vi "Template Write Parameter File.vi"(6 "Export?":bool, 8 "error in (no error)":errorcluster, 9 "Export Path (\"\")":path, 10 "Parameters (empty)":T3, 11 "Template Record":T1) -> (0 "error out":errorcluster, 2 "Template Record 2":T1, 3 "Files":T2)   [LabVIEW 2011]
uses:
  Addons/internet/utils/keyedarr.llb/Keyed Array.ctl
  Template Record.ctl
  <vilib>/Utility/config.llb/Write Key (String).vi
  <vilib>/Utility/config.llb/NI_LVConfig.lvlib
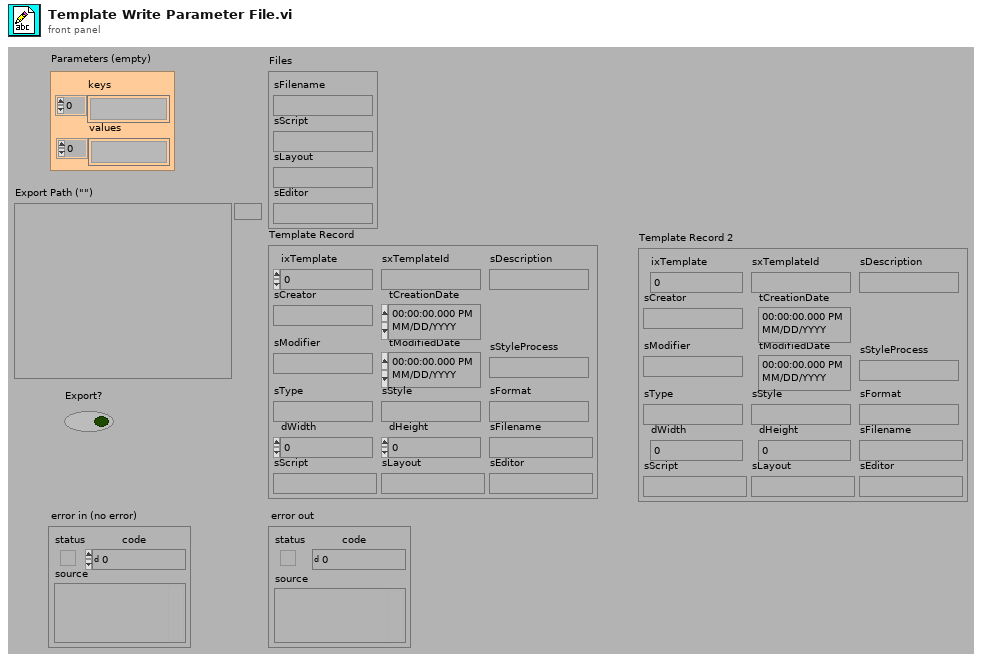
[diagram p1: front panel]
types:
  T1 = typedef "Template Record.ctl" = cluster{"ixTemplate":i32, "sxTemplateId":string, "sDescription":string, "sCreator":string, "tCreationDate":timestamp, "sModifier":string, "tModifiedDate":timestamp, "sType":string, "sStyle":string, "sFormat":string, "dWidth":dbl, "dHeight":dbl, "sFilename":string, "sScript":string, "sLayout":string, "sEditor":string, "sStyleProcess":string}
  T2 = cluster{"sFilename":string, "sScript":string, "sLayout":string, "sEditor":string}
  T3 = typedef "Keyed Array.ctl" = cluster{"keys":string[], "values":string[]}
  T4 = typedef "NI_LVConfig.lvlib/Config Data RefNum.ctl" = refnum<k1>
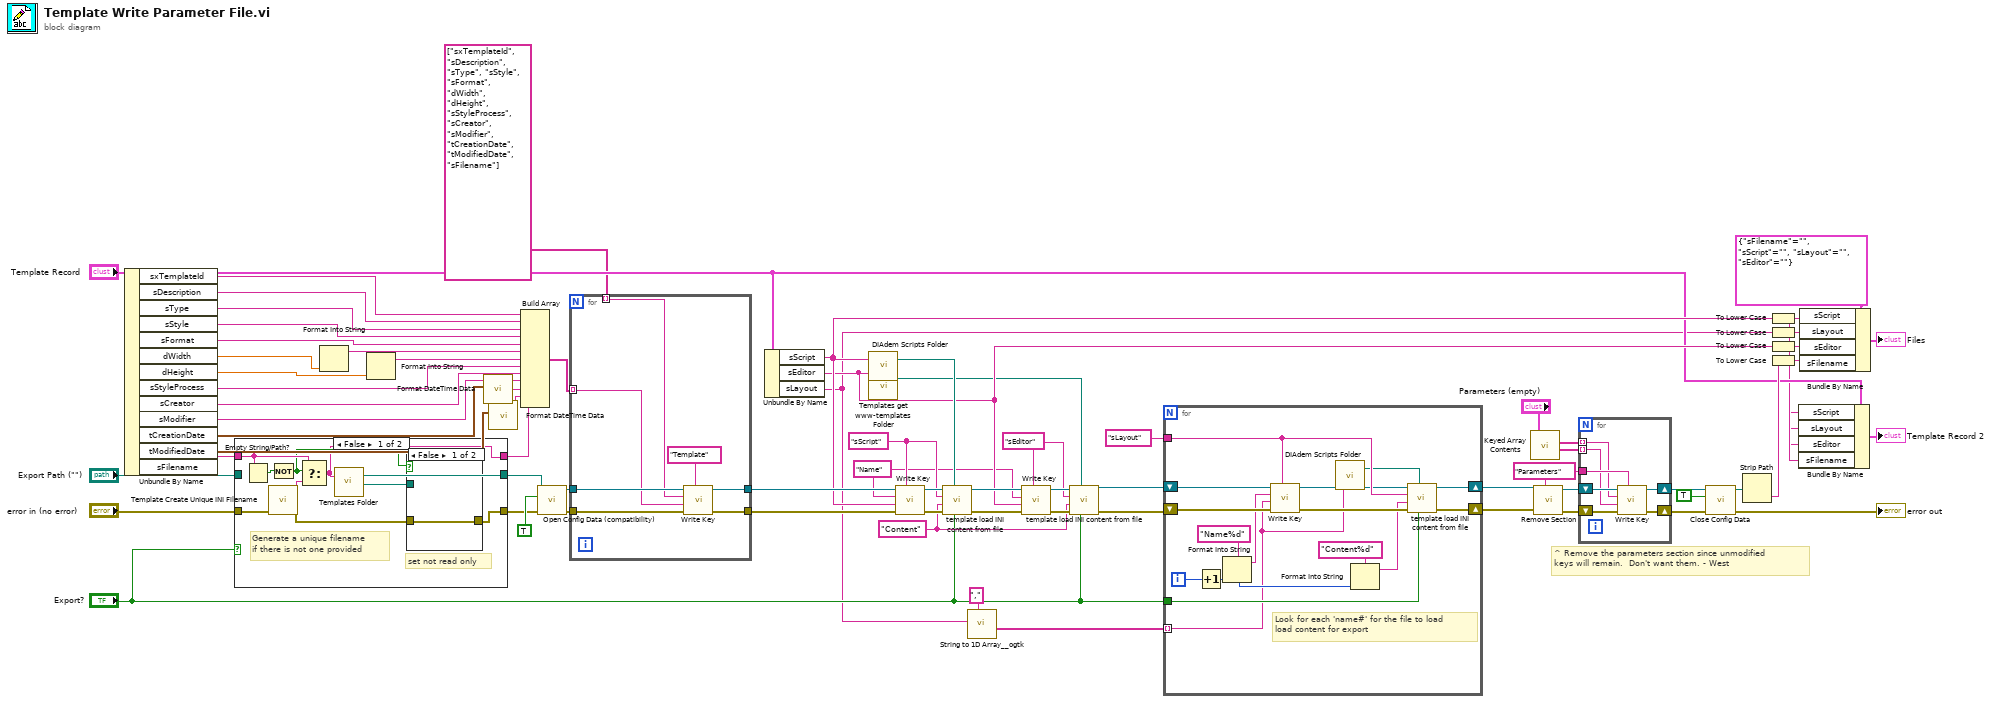
[diagram p0: block diagram]
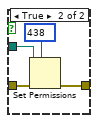
[diagram p2: hidden frame]
diagram:
  w29 = "Content" ("section")
  w40 = "Parameters" ("section")
  w32 = "sEditor" ("section")
  w28 = "Name" ("section")
  w37 = "sScript" ("section")
  # "^ Remove the parameters section since unmodified\nkeys will remain.  Don't want them. - West"
  n1 = Unbundle By Name("Template Record") -> ("sxTemplateId"=w67:string, "sDescription"=w65:string, "sType"=w64:string, "sStyle"=w63:string, "sFormat"=w41:string, "dWidth"=w47:dbl, "dHeight"=w45:dbl, "sStyleProcess"=w12:string, "sCreator"=w10:string, "sModifier"=w9:string, "tCreationDate"=w8:timestamp, "tModifiedDate"=w5:timestamp, "sFilename"=w62:string)
  n2 = case shown="False" "Export?" {
    tunnel: [w74 w89] -> w20
    tunnel: w62 -> [w80 w87]
    tunnel: "error in (no error)" -> [w78 w88]
    tunnel: [w76 w88] -> w13
    tunnel: "Export Path (\"\")" -> [_ w89]
    tunnel: [w73 w87] -> w4
    frame False {
      # "set not read only"
      # "Generate a unique filename\nif there is not one provided"
      n3 = Empty String/Path?(string/path=w80) -> (empty?=w81:bool)
      n4 = Not(x=w81) -> (.not. x?=w75:bool)
      n5 = call "Template Create Unique INI Filename.vi"("error in (no error)"=w78) -> ("error out"=w77:errorcluster, "INI Name"=w79:string)  [unwired: 9 out]
      n6 = Select(t=w80, s=w75, f=w79) -> (s? t:f=w73:string)
      n7 = call "Templates Folder.vi"("Relative Path (\"\")"=w73) -> ("Templates Folder"=w74:path)  [unwired: 2 out]
      n8 = case shown="False" w75 {
        tunnel: w77 -> [w82 w86]
        tunnel: [w82 w85] -> w76
        tunnel: w74 -> [_ w84]
        frame False {
        }
        frame True {
          n9 = Set Permissions(7:i16 438 ("permissions"), 8:w86, 11:w84) -> (0:w85:errorcluster)  [unwired: 3 out]
        }
      }
    }
    frame True {
    }
  }
  n10 = Format Into String(w47) -> (resulting string=w46:string)  [unwired: 3 in, 1 out]
  n11 = Format Into String(w45) -> (resulting string=w44:string)  [unwired: 3 in, 1 out]
  n12 = call "Format DateTime Data.vi"("Timestamp in"=w8) -> ("UTC DB String out"=w7:string)  [unwired: 10 out]
  n13 = call "Format DateTime Data.vi"("Timestamp in"=w5) -> ("UTC DB String out"=w6:string)  [unwired: 10 out]
  n14 = Build Array(w67, w65, w64, w63, w41, w46, w44, w12, w10, w9, w7, w6, w4) -> (w66:string[])
  n15 = call <vilib>:"Open Config Data (compatibility).vi"("error in (no error)"=w13, "create file if necessary (T)"=TRUE, "configuration file path"=w20) -> ("error out"=w69:errorcluster, "refnum"=w68:T4)  [unwired: 6 in, 1 out]
  n16 = for {
    tunnel: w69 -> [w96]
    tunnel: string[] ["sxTemplateId", "sDescription", "sType", "sStyle", "sFormat", "dWidth", "dHeight", "sStyleProcess", "sCreator", "sModifier", "tCreationDate", "tModifiedDate", "sFilename"] -> [w92] mode=indexing
    tunnel: [w95] -> w51
    tunnel: w68 -> [w94]
    tunnel: [w91] -> w52
    tunnel: w66 -> [w90] mode=indexing
    n17 = call-poly <vilib>:"Write Key.vi"("section"="Template", "error in (no error)"=w96, "value"=w90, "key"=w92, "refnum"=w94) -> ("error out"=w95:errorcluster, "refnum out"=w91:T4)  [unwired: 1 in, 4 out]
  }
  n18 = Unbundle By Name("Template Record") -> ("sScript"=w48:string, "sEditor"=w31:string, "sLayout"=w3:string)
  n19 = call "DIAdem Scripts Folder.vi"("Relative Path (\"\" - Folder)"=w48) -> ("Scripts Folder"=w38:path)  [unwired: 2 out]
  n20 = call "Templates get www-templates Folder.vi"("Relative Path (\"\")"=w31) -> ("WWW-templates Folder"=w30:path)  [unwired: 2 in]
  n21 = call-poly <vilib>:"Write Key.vi"("section"=w37, "error in (no error)"=w51, "value"=w48, "key"=w28, "refnum"=w52) -> ("error out"=w50:errorcluster, "refnum out"=w39:T4)  [unwired: 1 in, 4 out]
  n22 = call "template load INI content from file.vi"("Export?"="Export?", "FILE TO LOAD"=w38, "error in"=w50, "KEY"=w29, "section"=w37, "refnum out"=w39) -> ("error out"=w33:errorcluster, "refnum out 2"=w34:T4)  [unwired: 2 in, 2 out]
  n23 = call "String to 1D Array__ogtk.vi"("delimiter (Tab)"=",", "string"=w3) -> ("Array of Strings"=w2:string[])  [unwired: 9 in]
  n24 = call-poly <vilib>:"Write Key.vi"("section"=w32, "error in (no error)"=w33, "value"=w31, "key"=w28, "refnum"=w34) -> ("error out"=w35:errorcluster, "refnum out"=w36:T4)  [unwired: 1 in, 4 out]
  n25 = call "template load INI content from file.vi"("Export?"="Export?", "FILE TO LOAD"=w30, "error in"=w35, "KEY"=w29, "section"=w32, "refnum out"=w36) -> ("error out"=w26:errorcluster, "refnum out 2"=w25:T4)  [unwired: 2 in, 2 out]
  n26 = for {
    tunnel: "sLayout" ("section") -> [w111]
    shift-right: [w109] -> w23
    shift-left: w26 -> [w110]
    shift-right: [w108] -> w24
    shift-left: w25 -> [w112]
    tunnel: "Export?" -> [w107]
    tunnel: w2 -> [w97] mode=indexing
    i -> [w102]
    # "Look for each 'name#' for the file to load\nload content for export"
    n27 = Increment(x=w102) -> (x+1=w101:i32)
    n28 = Format Into String(format string="Name%d" ("section"), w101) -> (resulting string=w103:string)  [unwired: 2 in, 1 out]
    n29 = call-poly <vilib>:"Write Key.vi"("section"=w111, "error in (no error)"=w110, "value"=w97, "key"=w103, "refnum"=w112) -> ("error out"=w106:errorcluster, "refnum out"=w105:T4)  [unwired: 1 in, 4 out]
    n30 = call "DIAdem Scripts Folder.vi"("Relative Path (\"\" - Folder)"=w97) -> ("Scripts Folder"=w100:path)  [unwired: 2 out]
    n31 = Format Into String(format string="Content%d" ("section"), w101) -> (resulting string=w98:string)  [unwired: 2 in, 1 out]
    n32 = call "template load INI content from file.vi"("Export?"=w107, "FILE TO LOAD"=w100, "error in"=w106, "KEY"=w98, "section"=w111, "refnum out"=w105) -> ("error out"=w109:errorcluster, "refnum out 2"=w108:T4)  [unwired: 4 out]
  }
  n33 = call "Keyed Array Contents.vi"("array in"="Parameters (empty)") -> ("values"=w59:string[], "keys"=w60:string[])  [unwired: 5 out]
  n34 = call <vilib>:"Remove Section.vi"("section"=w40, "error in (no error)"=w23, "refnum"=w24) -> ("error out"=w42:errorcluster, "refnum out"=w43:T4)  [unwired: 7 out]
  n35 = for {
    shift-right: [w118] -> w54
    shift-left: w43 -> [w119]
    tunnel: w60 -> [w114] mode=indexing
    tunnel: w59 -> [w113] mode=indexing
    shift-right: [w116] -> w53
    shift-left: w42 -> [w117]
    tunnel: w40 -> [w115]
    n36 = call-poly <vilib>:"Write Key.vi"("section"=w115, "error in (no error)"=w117, "value"=w113, "key"=w114, "refnum"=w119) -> ("error out"=w116:errorcluster, "refnum out"=w118:T4)  [unwired: 1 in, 4 out]
  }
  n37 = call <vilib>:"Close Config Data.vi"("error in (no error)"=w53, "write file if changed (T)"=TRUE, "refnum"=w54) -> ("error out"=→"error out":errorcluster, "file path"=w55:path)  [unwired: 7 out]
  n38 = Strip Path(path=w55) -> (name=w57:string)  [unwired: 1 out]
  n39 = To Lower Case(string=w48) -> (all lower case string=w15:string)
  n40 = To Lower Case(string=w3) -> (all lower case string=w16:string)
  n41 = To Lower Case(string=w31) -> (all lower case string=w17:string)
  n42 = To Lower Case(string=w57) -> (all lower case string=w18:string)
  n43 = Bundle By Name(cluster="Template Record", "sScript"=w15, "sLayout"=w16, "sEditor"=w17, "sFilename"=w18) -> (→"Template Record 2":T1)
  n44 = Bundle By Name(cluster=T2 {"sFilename"="", "sScript"="", "sLayout"="", "sEditor"=""} ("Files"), "sScript"=w15, "sLayout"=w16, "sEditor"=w17, "sFilename"=w18) -> (→"Files":T2)
